vi "Manlight-Connection.vi"(4 "error in":errorcluster, 5 "Connect?":bool, 6 "VISA Refnum in":refnum<visa-resource-name>) -> (0 "error out":errorcluster, 1 "Status":string, 2 "VISA Refnum out":refnum<visa-resource-name>, 3 "Manlight Laser Connected":bool)   [LabVIEW 2020]
uses:
  <vilib>/Instr/_visa.llb/VISA Configure Serial Port (Instr).vi
  <vilib>/Instr/_visa.llb/Select Event Type.ctl
panel:
  in  "Intf Inst Name":string
  in  "regular expression":string="COM5"
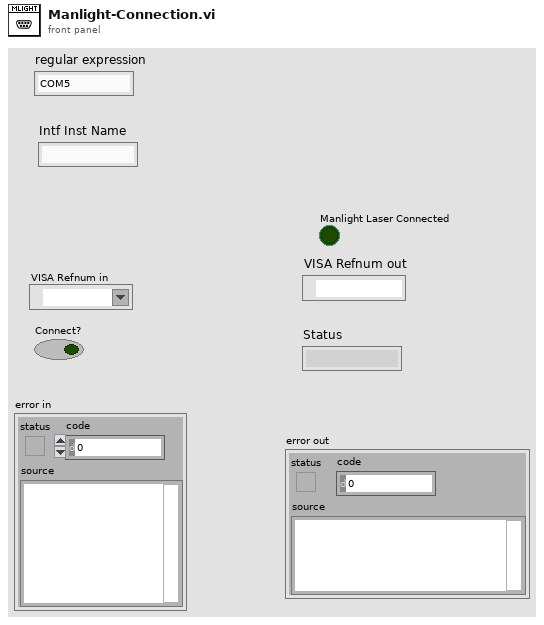
[diagram p1: front panel]
types:
  T1 = typedef "Select Event Type.ctl" = u32
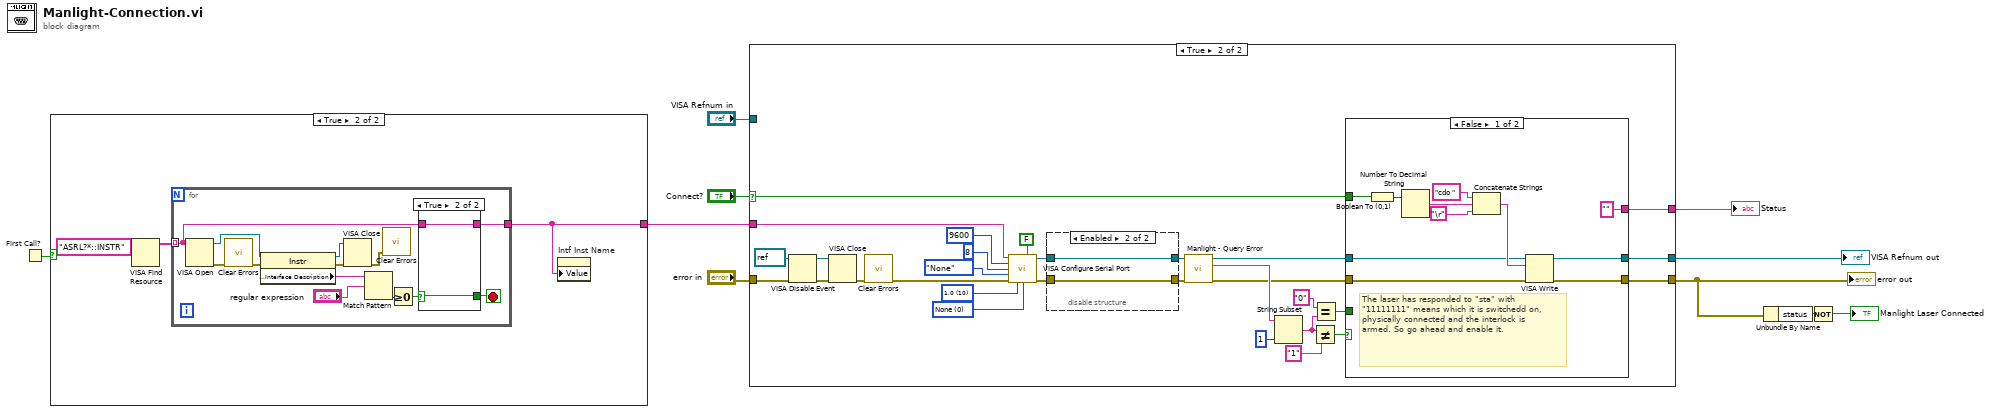
[diagram p0: block diagram]
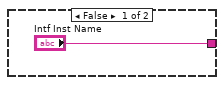
[diagram p2: hidden frame]
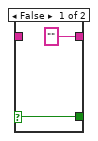
[diagram p3: hidden frame]
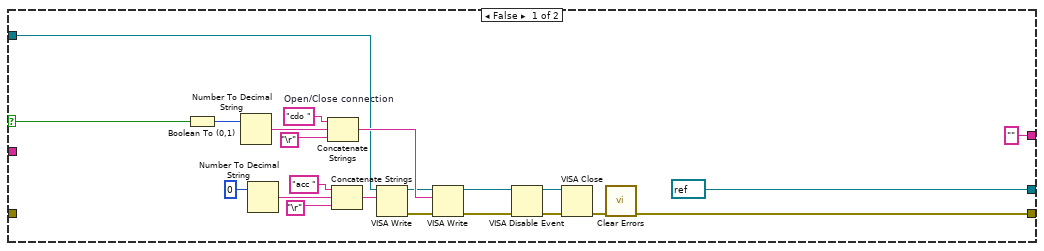
[diagram p4: hidden frame]
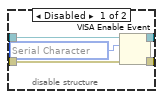
[diagram p5: hidden frame]
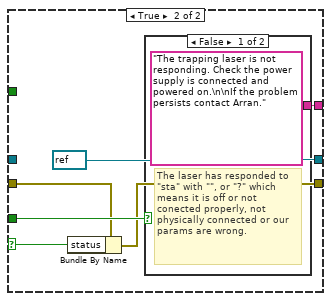
[diagram p6: hidden frame]
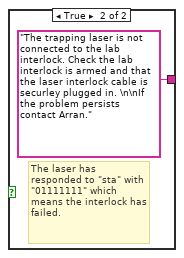
[diagram p7: hidden frame]
diagram:
  n1 = First Call?() -> (First Call?: T/F=w1:bool)
  n2 = case shown="True" w1 {
    tunnel: ["Intf Inst Name" w12] -> w5
    frame False {
    }
    frame True {
      n3 = VISA Find Resource(11:"ASRL?*::INSTR" ("expression (\"\")")) -> (3:w13:string[])  [unwired: 2 in, 2 out]
      n4 = for {
        tunnel: w13 -> [w16] mode=indexing
        tunnel: [w18] -> w12
        stop <- w19 stop-if-true
        n5 = VISA Open(VISA resource name=w16) -> (VISA resource name=w23:refnum<visa-resource-name>, error out=w26:errorcluster)  [unwired: 4 in]
        n6 = call <vilib>:"Clear Errors.vi"("error in (no error)"=w26) -> ("error out"=w22:errorcluster)  [unwired: 5 in, 1 out]
        n7 = property class="Instr"(reference=w23, error in=w22) -> (reference out=w27:refnum<visa-resource-name>, error out=w25:errorcluster, "Interface Information:Interface Description"=w20:string)
        n8 = VISA Close(VISA resource name=w27, error in (no error)=w25) -> (error out=w17:errorcluster)
        n9 = Match Pattern(string=w20, regular expression="regular expression") -> (offset past match=w15:i32)  [unwired: 1 in, 3 out]
        n10 = call <vilib>:"Clear Errors.vi"("error in (no error)"=w17) -> ()  [unwired: 5 in, 2 out]
        n11 = Greater Or Equal To 0?(x=w15) -> (x >= 0?=w21:bool)
        n12 = case shown="True" w21 {
          selector: w21 -> [w29 w31]
          tunnel: w16 -> [_ w30]
          tunnel: [w29 w31] -> w19
          tunnel: ["" ("Intf Inst Name") w30] -> w18
          frame False {
          }
          frame True {
          }
        }
      }
      n13 = property on="Intf Inst Name" class="Str"("Value"=w12) -> ()  [unwired: 2 in, 2 out]
    }
  }
  n14 = case shown="True" "Connect?" {
    selector: "Connect?" -> [w45 w80]
    tunnel: w5 -> [_ w54]
    tunnel: [w43 w79] -> w7
    tunnel: "error in" -> [_ w78]
    tunnel: "VISA Refnum in" -> [w33 _]
    tunnel: [refnum<visa-resource-name> refnum ("VISA Refnum out") w60] -> w3
    tunnel: ["" w55] -> w2
    frame False {
      w50 = "cdo "  # Open/Close connection
      n15 = Boolean To (0,1)(Boolean=w45) -> (0, 1=w46:i16)
      n16 = Number To Decimal String(number=w46) -> (decimal integer string=w49:string)  [unwired: 1 in]
      n17 = Number To Decimal String(number=0) -> (decimal integer string=w40:string)  [unwired: 1 in]
      n18 = Concatenate Strings(w50, w49, "\r") -> (w47:string)
      n19 = Concatenate Strings("acc ", w40, "\r") -> (w38:string)
      n20 = VISA Write(VISA resource name=w33, write buffer=w38) -> (VISA resource name out=w37:refnum<visa-resource-name>, error out=w36:errorcluster)  [unwired: 1 in, 1 out]
      n21 = VISA Write(VISA resource name=w37, write buffer=w47, error in (no error)=w36) -> (VISA resource name out=w44:refnum<visa-resource-name>, error out=w42:errorcluster)  [unwired: 1 out]
      n22 = VISA Disable Event(8:w42, 11:w44) -> (0:w51:errorcluster, 3:w53:refnum<visa-resource-name>)  [unwired: 2 in]
      n23 = VISA Close(VISA resource name=w53, error in (no error)=w51) -> (error out=w52:errorcluster)
      n24 = call <vilib>:"Clear Errors.vi"("error in (no error)"=w52) -> ("error out"=w43:errorcluster)  [unwired: 5 in, 1 out]
    }
    frame True {
      w77 = u16 0 items=["None", "XON/XOFF", "RTS/CTS", "XON/XOFF & RTS/CTS", "DTR/DSR", "XON/XOFF & DTR/DSR"] ("flow control (0:none)")
      w76 = u16 10 items=["1.0"=10, "1.5"=15, "2.0"=20] ("Stop Bits")
      n25 = VISA Disable Event(8:w78, 11:refnum<visa-resource-name> refnum ("VISA resource name")) -> (0:w62:errorcluster, 3:w64:refnum<visa-resource-name>)  [unwired: 2 in]
      n26 = VISA Close(VISA resource name=w64, error in (no error)=w62) -> (error out=w63:errorcluster)
      n27 = call <vilib>:"Clear Errors.vi"("error in (no error)"=w63) -> ("error out"=w81:errorcluster)  [unwired: 5 in, 1 out]
      n28 = call-poly "VISA Configure Serial Port"("VISA resource name"=w54, "Enable Termination\nChar (T)"=FALSE ("Enable Termination\nChar (T)"), "baud rate (9600)"=u32 9600, "data bits (8)"=u16 8 ("Data Bits"), "parity (0:none)"=enum16{"None", "Odd", "Even", "Mark", "Space"}."None" ("Parity"), "error in (no error)"=w81, "stop bits (10: 1 bit)"=w76, "flow control (0:none)"=w77) -> ("VISA resource name out"=w56:refnum<visa-resource-name>, "error out"=w83:errorcluster)  [unwired: 6 in]
      n29 = disable-structure shown="Enabled" {
        disable-tunnel: w83 -> [w88 w89]
        disable-tunnel: [w86 w89] -> w73
        disable-tunnel: [w85 w90] -> w57
        disable-tunnel: w56 -> [w84 w90]
        frame Disabled {
          w87 = T1 1073684533 items=["Service Request"=1073684491, "Trigger"=3221168138, "Clear"=1073684493, "VXI Signal"=1073684512, "VXI/VME Interrupt"=3221168161, "VXI/VME Sysfail"=1073684509, "VXI/VME Sysreset"=1073684510, "GPIB CIC"=1073684498, "GPIB Talk"=1073684499, "GPIB Listen"=1073684500, "PXI Interrupt"=1073684514, "Serial Break"=1073684515, "Serial TermChar"=1073684516, "Serial CTS"=1073684521, "Serial DSR"=1073684522, "Serial DCD"=1073684524, "Serial RI"=1073684526, "Serial Character"=1073684533, "USB Interrupt"=1073684535, "All Enabled"=1073709055] ("Event Type")
          n30 = VISA Enable Event(8:w88, 10:w87, 11:w84) -> (0:w86:errorcluster, 3:w85:refnum<visa-resource-name>)  [unwired: 1 in]
        }
        frame Enabled {
        }
      }
      n31 = call "Manlight - Query Error.vi"("error in (no error)"=w73, "VISA Refnum in"=w57) -> ("error out"=w69:errorcluster, "Error Status"=w72:string, "VISA Refnum out"=w58:refnum<visa-resource-name>)  [unwired: 7 in]
      n32 = String Subset(string=w72, length (rest)=1 ("length (rest)")) -> (substring=w66:string)  [unwired: 1 in]
      n33 = Not Equal?(x=w66, y="1") -> (x != y?=w70:bool)
      n34 = Equal?(x="0", y=w66) -> (x = y?=w67:bool)
      n35 = case shown="False" w70 {
        selector: w70 -> [_ w105]
        tunnel: w80 -> [w99 _]
        tunnel: [w98 w104] -> w79
        tunnel: [w96 refnum<visa-resource-name> refnum ("VISA Refnum out")] -> w60
        tunnel: w58 -> [w93 _]
        tunnel: w69 -> [w92 w106]
        tunnel: w67 -> [_ w107]
        tunnel: ["" w102] -> w55
        frame False {
          # "The laser has responded to \"sta\" with \"11111111\" means which it is switchedd on, physically connected and the interlock is armed. So go ahead and enable it."
          n36 = Boolean To (0,1)(Boolean=w99) -> (0, 1=w100:i16)
          n37 = Number To Decimal String(number=w100) -> (decimal integer string=w95:string)  [unwired: 1 in]
          n38 = Concatenate Strings("cdo ", w95, "\r") -> (w97:string)
          n39 = VISA Write(VISA resource name=w93, write buffer=w97, error in (no error)=w92) -> (VISA resource name out=w96:refnum<visa-resource-name>, error out=w98:errorcluster)  [unwired: 1 out]
        }
        frame True {
          n40 = Bundle By Name(cluster=w106, "status"=w105) -> (w104:errorcluster)
          n41 = case shown="False" w107 {
            tunnel: ["The trapping laser is not responding. Check the power supply is connected and powered on.\n\nIf the problem persists contact Arran." "The trapping laser is not connected to the lab interlock. Check the lab interlock is armed and that the laser interlock cable is securley plugged in. \n\nIf the problem persists contact Arran."] -> w102
            frame False {
              # "The laser has responded to \"sta\" with \"\", or \"?\" which means it is off or not conected properly, not physically connected or our params are wrong."
            }
            frame True {
              # "The laser has responded to \"sta\" with \"01111111\" which means the interlock has failed."
            }
          }
        }
      }
    }
  }
  "error out" <- w7
  "VISA Refnum out" <- w3
  "Status" <- w2
  n42 = Unbundle By Name(w7) -> ("status"=w8:bool)
  n43 = Not(x=w8) -> (.not. x?=→"Manlight Laser Connected":bool)
